vi "Set VDD Voltage and MeasV_w_Delay_No Data log.vi"(0 "Semiconductor Module Context":T1, 2 "Delay_after_Power_Up":dbl=0.001 format="%#_13p", 5 "Pins":string[](array[string])=["VDD"], 9 "VDD voltage level":dbl=1.8 caption="voltage level" format="%_6p", 11 "error in (no error)":errorcluster) -> (4 "Semiconductor Module Context Out":T1, 6 "Instrument Sessions Out":refnum<k15>[](array[refnum]), 15 "error out":errorcluster)   [LabVIEW 2013]
uses:
  <vilib>/NI_TestStand_SemiconductorModule/NI_TestStand_Semiconductor_Module.lvlibp/PinMap/General/SemiconductorModuleContext.ctl
  <vilib>/NI_TestStand_SemiconductorModule/NI_TestStand_Semiconductor_Module.lvlibp/PinMap/DC Power/PinsToNIDCPowerSessions.vi
  <vilib>/NI_TestStand_SemiconductorModule/NI_TestStand_Semiconductor_Module.lvlibp
panel:
  out "voltage measurements":dbl[][](array[numeric])
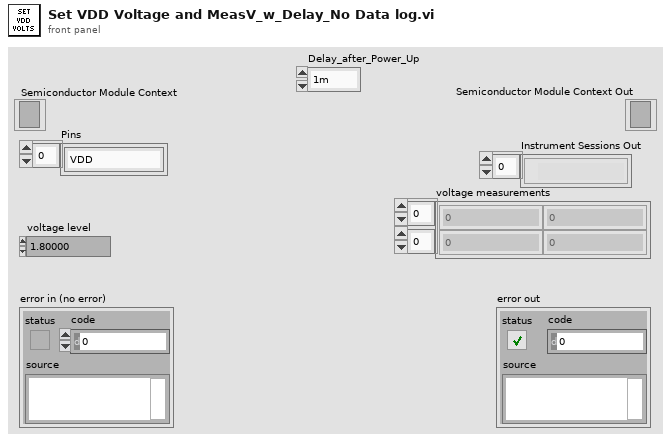
[diagram p1: front panel]
types:
  T1 = typedef "NI_TestStand_Semiconductor_Module.lvlibp/SemiconductorModuleContext.ctl" = refnum<k7>
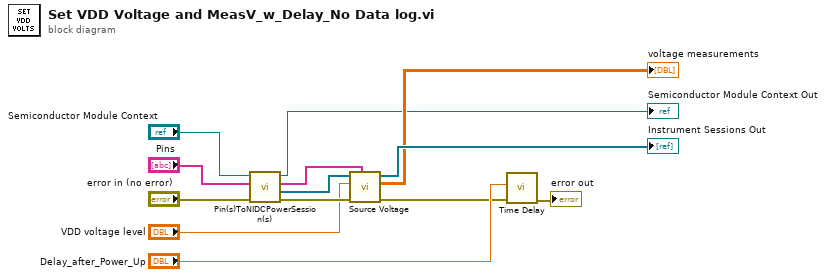
[diagram p0: block diagram]
diagram:
  n1 = call-poly <vilib>:"Pin(s)ToNIDCPowerSession(s).vi"("error in (no error)"="error in (no error)", "Pins"="Pins", "Semiconductor Module Context"="Semiconductor Module Context") -> ("error out"=w11:errorcluster, "Instrument Sessions"=w10:refnum<k15>[], "Channel Lists"=w4:string[], "Semiconductor Module Context Out"=→"Semiconductor Module Context Out":T1)  [unwired: 4 in, 1 out]
  n2 = call "Source Voltage.vi"("Channel Lists"=w4, "error in (no error)"=w11, "voltage level"="VDD voltage level", "Instrument Sessions In"=w10) -> ("error out"=w2:errorcluster, "voltage measurements"=→"voltage measurements":dbl[][], "Instrument Sessions Out"=→"Instrument Sessions Out":refnum<k15>[])  [unwired: 4 in, 1 out]
  n3 = call "Time Delay"("error in (no error)"=w2, "Delay Time (s)"="Delay_after_Power_Up") -> ("error out"=→"error out":errorcluster)  [unwired: 9 in]
